vi "Module Type.vi"(11 "Timing Module in":refnum<class "Timing Module.lvclass">) -> (2 "Module Type":string)   [LabVIEW 2020, in "Volatus.lvlib" / "Timing Module.lvclass"]
uses:
  Timing Module.lvclass
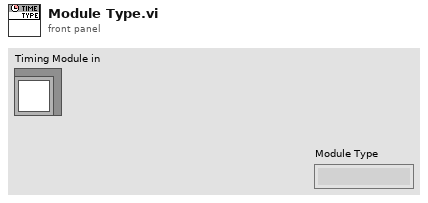
[diagram p1: front panel]
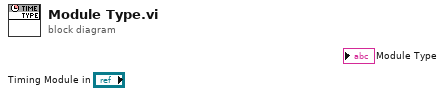
[diagram p0: block diagram]
diagram:
